vi "二位数组.vi"(3 "二位数组（输入）":dbl[][](array[numeric])) -> (0 "Numeric":dbl, 1 "字符串（输出）":string)   [LabVIEW 2018]
uses:
  <vilib>/Utility/error.llb/whitespace.ctl
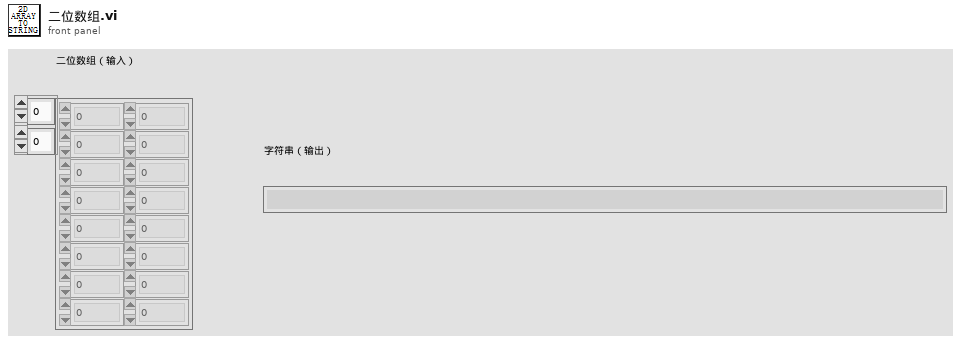
[diagram p1: front panel]
types:
  T1 = typedef "whitespace.ctl" = u16
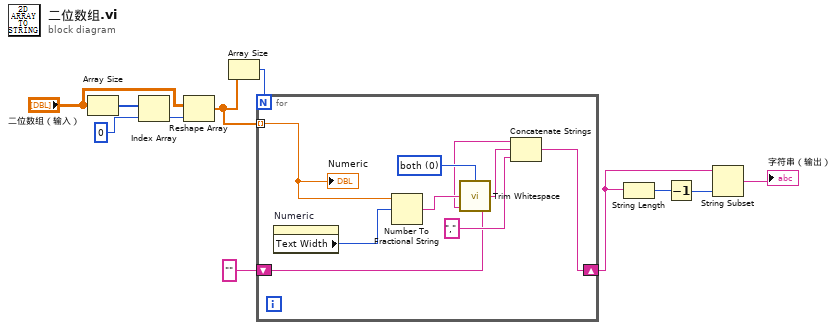
[diagram p0: block diagram]
diagram:
  n1 = Array Size(array="二位数组（输入）") -> (size(s)=w1:i32[])
  n2 = Index Array(array=w1, index=0 ("index (row)")) -> (element=w3:i32)
  n3 = Reshape Array("二位数组（输入）", w3) -> (w10:dbl[])
  n4 = Array Size(array=w10) -> (size(s)=w4:i32)
  n5 = for {
    N: w4 -> [_]
    tunnel: w10 -> [w19] mode=indexing
    shift-right: [w15] -> w11
    shift-left: "" -> [w12]
    w17 = T1 0 items=["both", "start of string", "end of string"] ("location (both)")
    n6 = property on="Numeric" class="DigNum (严格)"() -> ("Text Width"=w13:u32)  [unwired: 2 in, 2 out]
    n7 = Number To Fractional String(number=w19, width (-)=w13) -> (F-format string=w18:string)  [unwired: 2 in]
    n8 = call <vilib>:"Trim Whitespace.vi"("string"=w18, "location (both)"=w17) -> ("trimmed string"=w14:string)
    n9 = Concatenate Strings(w12, w14, ",") -> (w15:string)
    "Numeric" <- w19
  }
  n10 = String Length(string=w11) -> (length=w6:i32)
  n11 = Decrement(x=w6) -> (x-1=w7:i32)
  n12 = String Subset(string=w11, length (rest)=w7) -> (substring=→"字符串（输出）":string)  [unwired: 1 in]
